vi "Record in TXT silar.vi"(0 "Кол-во циклов":i32=1, 1 "Кол-во используемых растворов":i32(ring)=4 items=["Один"=1, "Два"=2, "Три"=3, "Четыре"=4], 2 "Кол-во погружений в каждый стакан":i32[](array[numeric])=[1, 1, 1, 1], 3 "Опускания подложки в растворе":dbl[](array[numeric])=[1.0, 1.0, 1.0, 1.0], 4 "Глубина погружения в раствор [мм]":dbl[](array[numeric])=[20.0, 20.0, 20.0, 20.0], 5 "Опускания подложки до раствора":dbl[](array[numeric])=[2.9, 2.9, 2.9, 2.9], 6 "Режим погружения подложки":u16(ring) items=["Частичный", "Полный"], 7 "Высота подложки [мм]":dbl=25.0 format="%#3_3g", 8 "Подъема подложки над раствором":dbl[](array[numeric])=[2.9, 2.9, 2.9, 2.9], 9 "Кол-во жидкости в каждом стакане [мл]":dbl[](array[numeric])=[50.0, 50.0, 50.0, 50.0], 10 "Подъема подложки из раствора":dbl[](array[numeric])=[1.0, 1.0, 1.0, 1.0], 11 "Оператор":string="Андронов", 12 "Нахождения в растворе":dbl[](array[numeric])=[1.0, 1.0, 1.0, 1.0] caption="Время нахождения в растворе (секунды)", 13 "Получаемый образец":string="PbS", 14 "Высота стакана [мм]":dbl=81.2, 15 "Задержки после подъема из раствора":dbl[](array[numeric])=[0.0, 0.0, 0.0, 0.0], 17 "Необходимая температура":dbl[](array[numeric])=[0.0, 0.0, 0.0, 0.0], 19 "Все время процесса":timestamp=timestamp(-14394 s since 1904-01-01) format="%<%H:%M:%S>T") -> ()   [LabVIEW 2016]
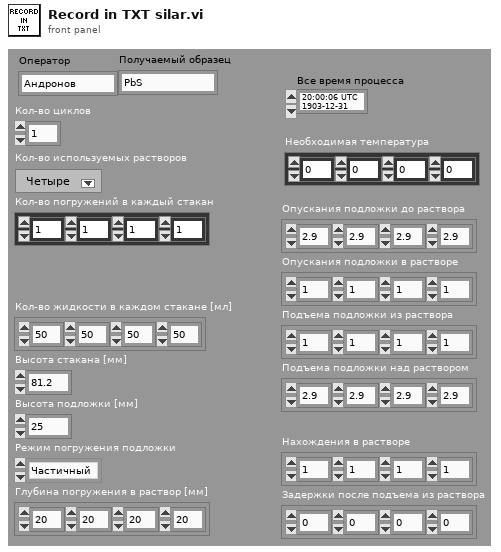
[diagram p1: front panel]
types:
  T1 = enum16{"open", "replace", "create", "open or create", "replace or create", "replace or create with confirmation"}
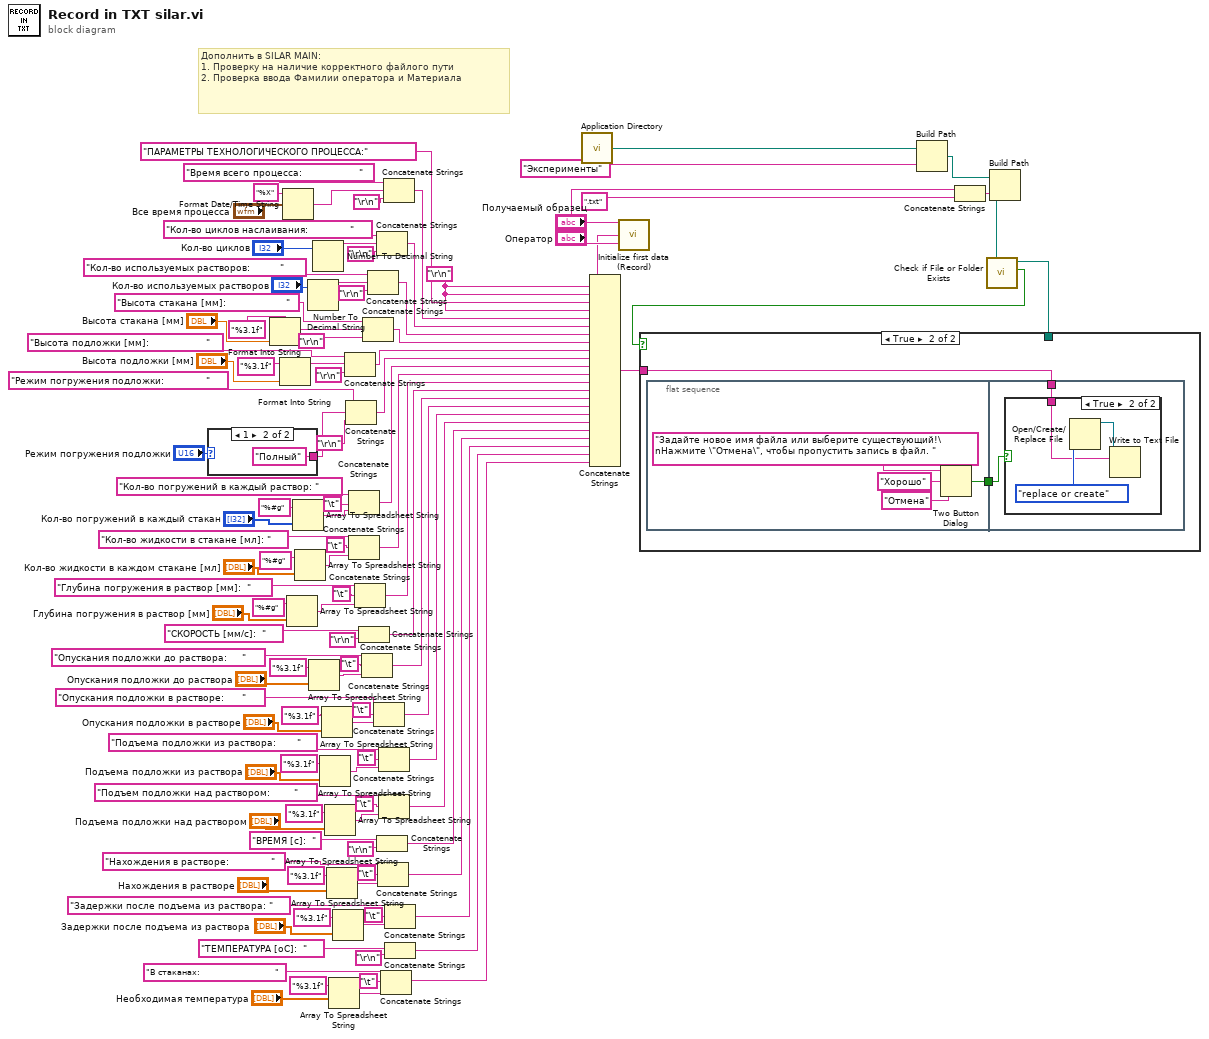
[diagram p0: block diagram]
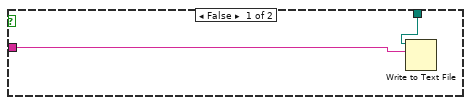
[diagram p2: hidden frame]
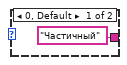
[diagram p4: hidden frame]
diagram:
  w58 = "\r\n"
  # "Дополнить в SILAR MAIN:\n1. Проверку на наличие корректного файлого пути\n2. Проверка ввода Фамилии оператора и Материала"
  n1 = case shown="1" "Режим погружения подложки" {
    tunnel: ["Частичный" "Полный"] -> w35
    frame 0, Default {
    }
    frame 1 {
    }
  }
  n2 = Format Into String(format string="%3.1f", "Высота стакана [мм]") -> (resulting string=w12:string)  [unwired: 2 in, 1 out]
  n3 = Format Into String(format string="%3.1f", "Высота подложки [мм]") -> (resulting string=w9:string)  [unwired: 2 in, 1 out]
  n4 = Format Date/Time String(time format string (%c)="%X", seconds (now)="Все время процесса") -> (date/time string=w55:string)  [unwired: 1 in]
  n5 = Array To Spreadsheet String(array="Глубина погружения в раствор [мм]", 3:"%#g" ("format (%.3f)")) -> (spreadsheet string=w92:string)  [unwired: 1 in]
  n6 = Array To Spreadsheet String(array="Кол-во погружений в каждый стакан", 3:"%#g" ("format (%.3f)")) -> (spreadsheet string=w95:string)  [unwired: 1 in]
  n7 = Array To Spreadsheet String(array="Кол-во жидкости в каждом стакане [мл]", 3:"%#g" ("format (%.3f)")) -> (spreadsheet string=w51:string)  [unwired: 1 in]
  n8 = Number To Decimal String(number="Кол-во используемых растворов") -> (decimal integer string=w97:string)  [unwired: 1 in]
  n9 = Array To Spreadsheet String(array="Опускания подложки до раствора", 3:"%3.1f" ("format (%.3f)")) -> (spreadsheet string=w87:string)  [unwired: 1 in]
  n10 = Number To Decimal String(number="Кол-во циклов") -> (decimal integer string=w100:string)  [unwired: 1 in]
  n11 = Array To Spreadsheet String(array="Подъема подложки из раствора", 3:"%3.1f" ("format (%.3f)")) -> (spreadsheet string=w81:string)  [unwired: 1 in]
  n12 = Array To Spreadsheet String(array="Опускания подложки в растворе", 3:"%3.1f" ("format (%.3f)")) -> (spreadsheet string=w83:string)  [unwired: 1 in]
  n13 = Array To Spreadsheet String(array="Подъема подложки над раствором", 3:"%3.1f" ("format (%.3f)")) -> (spreadsheet string=w79:string)  [unwired: 1 in]
  n14 = Array To Spreadsheet String(array="Нахождения в растворе", 3:"%3.1f" ("format (%.3f)")) -> (spreadsheet string=w77:string)  [unwired: 1 in]
  n15 = Array To Spreadsheet String(array="Необходимая температура", 3:"%3.1f" ("format (%.3f)")) -> (spreadsheet string=w73:string)  [unwired: 1 in]
  n16 = Array To Spreadsheet String(array="Задержки после подъема из раствора", 3:"%3.1f" ("format (%.3f)")) -> (spreadsheet string=w75:string)  [unwired: 1 in]
  n17 = Concatenate Strings("Высота подложки [мм]:                   " ("string"), w9, "\r\n") -> (w21:string)
  n18 = Concatenate Strings("Режим погружения подложки:              " ("string"), w35, "\r\n") -> (w20:string)
  n19 = Concatenate Strings("Кол-во погружений в каждый раствор: " ("string"), "\t", w95) -> (w19:string)
  n20 = Concatenate Strings("Кол-во жидкости в стакане [мл]: " ("string"), "\t", w51) -> (w18:string)
  n21 = Concatenate Strings("Глубина погружения в раствор [мм]:  " ("string"), "\t", w92) -> (w91:string)
  n22 = Concatenate Strings("СКОРОСТЬ [мм/c]:  " ("string"), "\r\n") -> (w86:string)
  n23 = Concatenate Strings("Опускания подложки до раствора:     " ("string"), "\t", w87) -> (w85:string)
  n24 = Concatenate Strings("Высота стакана [мм]:                    " ("string"), w12, "\r\n") -> (w22:string)
  n25 = Concatenate Strings("Кол-во используемых растворов:          " ("string"), w97, "\r\n") -> (w96:string)
  n26 = Concatenate Strings("Опускания подложки в растворе:      " ("string"), "\t", w83) -> (w68:string)
  n27 = Concatenate Strings("Кол-во циклов наслаивания:              " ("string"), w100, "\r\n") -> (w98:string)
  n28 = Concatenate Strings("ВРЕМЯ [c]:  " ("string"), "\r\n") -> (w65:string)
  n29 = Concatenate Strings("Нахождения в растворе:              " ("string"), "\t", w77) -> (w64:string)
  n30 = Concatenate Strings("Подъема подложки из раствора:       " ("string"), "\t", w81) -> (w67:string)
  n31 = Concatenate Strings("Подъем подложки над раствором:        " ("string"), "\t", w79) -> (w66:string)
  n32 = Concatenate Strings("В стаканах:                         " ("string"), "\t", w73) -> (w61:string)
  n33 = Concatenate Strings("Время всего процесса:                   " ("string"), w55, "\r\n") -> (w99:string)
  n34 = Concatenate Strings("Задержки после подъема из раствора: " ("string"), "\t", w75) -> (w63:string)
  n35 = Concatenate Strings("ТЕМПЕРАТУРА [oC]:  " ("string"), "\r\n") -> (w62:string)
  n36 = call <vilib>:"Application Directory.vi"() -> ("Application Directory"=w3:path)
  n37 = call "Initialize first data (Record).vi"("Оператор"="Оператор", "Получаемый материал"="Получаемый образец") -> ("Выходные данные"=w13:string)
  n38 = Concatenate Strings(w13, w58, w58, "ПАРАМЕТРЫ ТЕХНОЛОГИЧЕСКОГО ПРОЦЕССА:" ("string"), w58, w99, w98, w96, w22, w21, w20, w19, w18, w91, w86, w85, w68, w67, w66, w65, w64, w63, w62, w61) -> (w101:string)
  n39 = Build Path(base path=w3, name or relative path="Эксперименты") -> (appended path=w1:path)
  n40 = Concatenate Strings("Получаемый образец", ".txt" ("string")) -> (w16:string)
  n41 = Build Path(base path=w1, name or relative path=w16) -> (appended path=w6:path)
  n42 = call <vilib>:"Check if File or Folder Exists.vi"("path"=w6) -> ("file or folder exists?"=w5:bool, "dup path"=w4:path)  [unwired: 8 in, 1 out]
  n43 = case shown="True" w5 {
    tunnel: w101 -> [w119 w122]
    tunnel: w4 -> [w120 _]
    frame False {
      n44 = Write to Text File(file (use dialog)=w120, text=w119) -> ()  [unwired: 2 in, 3 out]
    }
    frame True {
      n45 = flat-sequence {
        tunnel: [w123] -> w121
        tunnel: w122 -> [w128]
        tunnel: w121 -> [w127]
        frame #0 {
          n46 = Two Button Dialog(message="Задайте новое имя файла или выберите существующий!\nНажмите \"Отмена\", чтобы пропустить запись в файл. ", 1:"Отмена" ("F button name (\"Cancel\")"), 2:"Хорошо" ("T button name (\"OK\")")) -> (T button?=w123:bool)
        }
        frame #1 {
          n47 = case shown="True" w127 {
            tunnel: w128 -> [_ w129]
            frame False {
            }
            frame True {
              n48 = Open/Create/Replace File(operation (0:open)=T1."replace or create") -> (refnum out=w130:refnum<file>)  [unwired: 5 in, 2 out]
              n49 = Write to Text File(file (use dialog)=w130, text=w129) -> ()  [unwired: 2 in, 3 out]
            }
          }
        }
      }
    }
  }
